vi "LVClass_CameraSet ctor.vi"(0 "CameraSet (const)":refnum<class "CameraSet.lvclass">, 5 "Configuration file path":path, 11 "error in (no error)":errorcluster) -> (4 "CameraSet (new)":refnum<class "CameraSet.lvclass">, 15 "error out":errorcluster)   [LabVIEW 2020, in "CameraSet.lvclass"]
doc: "CameraSet constructor.\n\n<B>camera_setIn</B> : Constant Pointer to CameraSet object.\n<B>camera_setOut</B> : Constant Pointer to CameraSet object.\n<B>config_file_path</B> : Absolute path to Haso or Camera configuration file."
uses:
  CameraSet.lvclass
  Handle creation.ctl
  CameraSet.lvclass/CameraSet.ctl
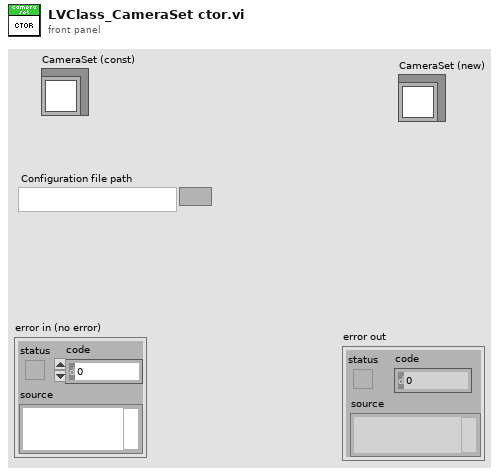
[diagram p1: front panel]
types:
  T1 = typedef "Handle creation.ctl" = enum16{"By ctor", "By write function"}
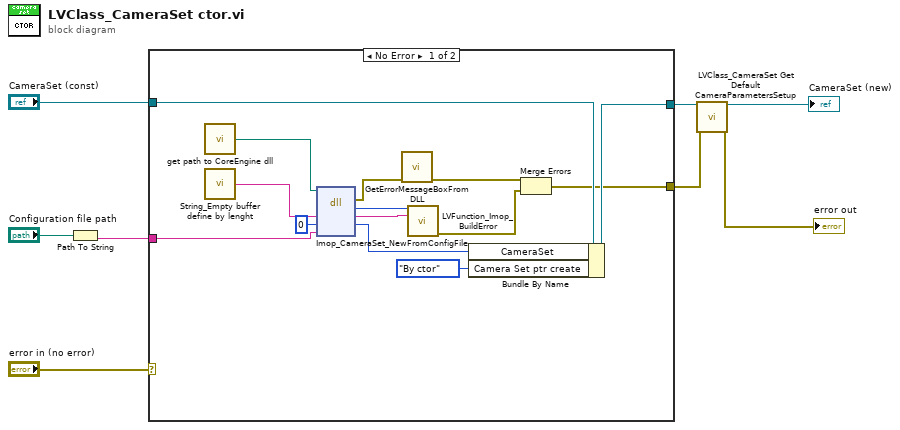
[diagram p0: block diagram]
diagram:
  n1 = Path To String(path="Configuration file path") -> (string=w6:string)
  n2 = case shown="No Error" "error in (no error)" {
    selector: "error in (no error)" -> [_ w23]
    tunnel: w6 -> [w17 _]
    tunnel: "CameraSet (const)" -> [w16 w24]
    tunnel: [w15 w24] -> w3
    tunnel: [w9 w23] -> w1
    frame No Error {
      n3 = call "get path to CoreEngine dll.vi"() -> ("path to wavekit library"=w14:path)  [unwired: 14 in, 1 out]
      n4 = call "String_Empty buffer define by lenght.vi"() -> ("Empty buffer"=w22:string)  [unwired: 1 in]
      n5 = dll-call lib="D:/soft/HASO_v3/SVN_trunk/ImOpCoreEngine4_LV2011/DLLs/c_interface_vc100.dll" fn="Imop_CameraSet_NewFromConfigFile"(path in=w14, "message"=w22, "objet"=0, "chemin_config"=w17) -> (error out=w13:errorcluster, "return type"=w19:i32, "message"=w20:string, "objet"=w21:i64)  [unwired: 3 in, 1 out]
      n6 = call "GetErrorMessageBoxFromDLL.vi"("error IN"=w13) -> ("error OUT"=w11:errorcluster)  [unwired: 10 in]
      n7 = call "LVFunction_Imop_BuildError.vi"("code"=w19, "String to Prepend to source (\"\")"=w20) -> ("error out"=w10:errorcluster)  [unwired: 13 in]
      n8 = Bundle By Name(cluster=w16, "CameraSet"=w21, "Camera Set ptr create"=Handle_creation."By ctor") -> (w15:refnum<class "CameraSet.lvclass">)
      n9 = Merge Errors(w11, w10) -> (w9:errorcluster)
    }
    frame Error {
    }
  }
  n10 = call "LVClass_CameraSet Get Default CameraParametersSetup.vi"("CameraSet in"=w3, "error in (no error)"=w1) -> ("CameraSet out"=→"CameraSet (new)":refnum<class "CameraSet.lvclass">, "error out"=→"error out":errorcluster)  [unwired: 9 in, 3 out]
